vi "CheckArraySize.vi"() -> ()   [LabVIEW 2011]
uses:
  <vilib>/Utility/error.llb/DialogType.ctl
panel:
  out "error out":errorcluster
  out "Numeric Indicator 3":dbl
  out "Numeric Indicator 2":dbl
  out "Numeric Indicator":dbl
  in  "Array 3":bool[](array[boolean])
  in  "Array 2":string[](array[string])
  in  "Array":string[](array[string])
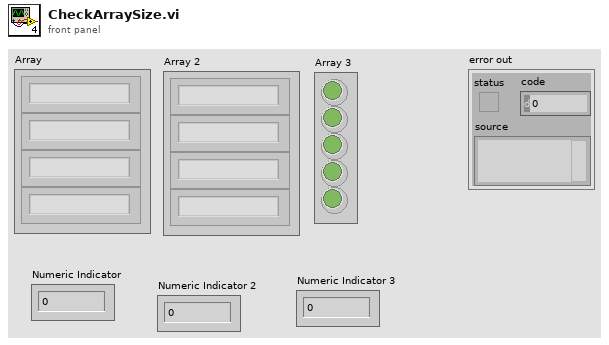
[diagram p1: front panel]
types:
  T1 = typedef "DialogType.ctl" = u16
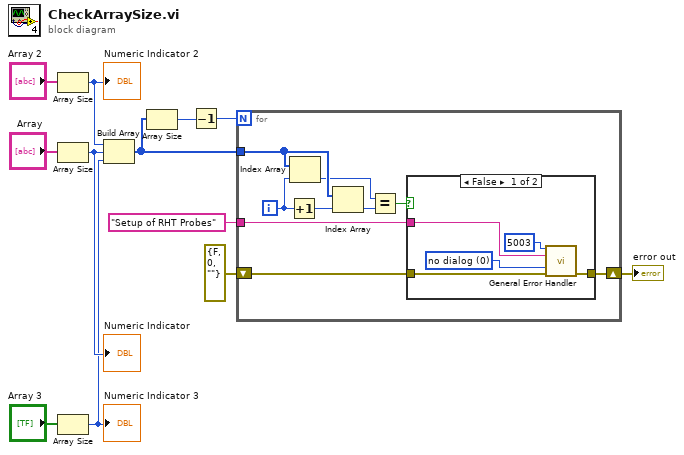
[diagram p0: block diagram]
diagram:
  n1 = Array Size(array="Array 2") -> (size(s)=w4:i32)
  "Numeric Indicator 2" <- w4
  n2 = Array Size(array="Array") -> (size(s)=w5:i32)
  "Numeric Indicator" <- w5
  n3 = Array Size(array="Array 3") -> (size(s)=w3:i32)
  "Numeric Indicator 3" <- w3
  n4 = Build Array(w4, w5, w3) -> (w12:i32[])
  n5 = Array Size(array=w12) -> (size(s)=w11:i32)
  n6 = Decrement(x=w11) -> (x-1=w10:i32)
  n7 = for {
    N: w10 -> [_]
    tunnel: w12 -> [w21]
    tunnel: "Setup of RHT Probes" ("[error source] (\" \")") -> [w13]
    shift-right: [w14] -> w1
    shift-left: errorcluster {"status"=FALSE, "code"=0, "source"=""} ("error constant") -> [w15]
    i -> [w19]
    n8 = Increment(x=w19) -> (x+1=w20:i32)
    n9 = Index Array(array=w21, index=w19) -> (element=w18:i32)
    n10 = Index Array(array=w21, index=w20) -> (element=w17:i32)
    n11 = Equal?(x=w18, y=w17) -> (x = y?=w16:bool)
    n12 = case shown="False" w16 {
      tunnel: w15 -> [w26 w27]
      tunnel: [w25 w27] -> w14
      tunnel: w13 -> [w22 _]
      frame False {
        w24 = T1 0 items=["no dialog", "OK message", "continue or stop message", "OK message + warnings", "continue/stop + warnings"] ("type of dialog (OK msg:1)")
        n13 = call <vilib>:"General Error Handler.vi"("[error code] (0)"=5003, "[error source] (\" \")"=w22, "type of dialog (OK msg:1)"=w24, "error in (no error)"=w26) -> ("error out"=w25:errorcluster)  [unwired: 7 in, 4 out]
      }
      frame True {
      }
    }
  }
  "error out" <- w1
